vi "create.vi"(8 "error in":errorcluster, 10 "devices":refnum<class "test-device.lvclass">[](array[class]), 11 "test-system in":refnum<class "test-system.lvclass">) -> (0 "error out":errorcluster, 3 "test-system out":refnum<class "test-system.lvclass">)   [LabVIEW 2020, in "test-system.lvclass"]
uses:
  test-system.lvclass
  test-device/test-device.lvclass
  test-system.lvclass/test-system.ctl
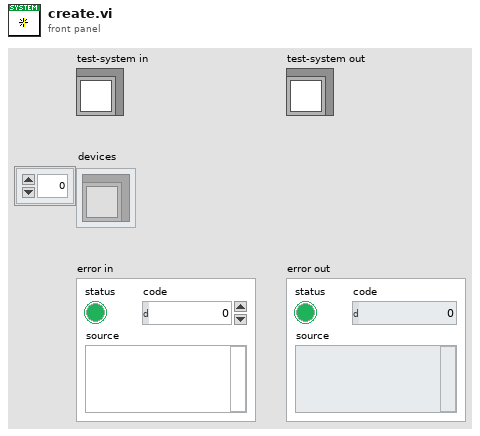
[diagram p1: front panel]
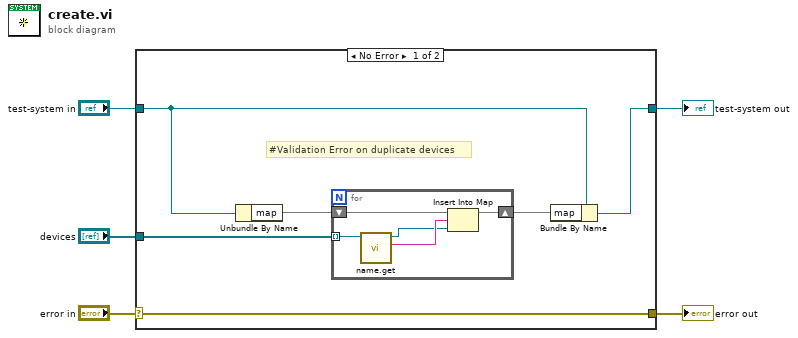
[diagram p0: block diagram]
diagram:
  n1 = case shown="No Error" "error in" {
    selector: "error in" -> [w11 w18]
    tunnel: [w11 w18] -> w4
    tunnel: [w8 w17] -> w2
    tunnel: "test-system in" -> [w7 w17]
    tunnel: "devices" -> [w6 _]
    frame No Error {
      # "#Validation Error on duplicate devices"
      n2 = Unbundle By Name(w7) -> ("map"=w9:map{string, refnum<class "test-device.lvclass">})
      n3 = for {
        shift-right: [w15] -> w10
        shift-left: w9 -> [w14]
        tunnel: w6 -> [w13] mode=indexing
        n4 = call "name.get.vi"("test-device in"=w13) -> ("name"=w16:string, "test-device out"=w12:refnum<class "test-device.lvclass">)  [unwired: 9 in]
        n5 = Insert Into Map(map in=w14, key=w16, value=w12) -> (map out=w15:map{string, refnum<class "test-device.lvclass">})  [unwired: 2 out]
      }
      n6 = Bundle By Name(cluster=w7, "map"=w10) -> (w8:refnum<class "test-system.lvclass">)
    }
    frame Error {
    }
  }
  "error out" <- w4
  "test-system out" <- w2
